vi "Create.vi"(5 "StringContains In":refnum<class "StringContains.lvclass">, 7 "Ignore Case (F)":bool, 8 "error in (no error)":errorcluster, 10 "Needle":string) -> (0 "error out":errorcluster, 3 "StringContains":refnum<class "StringContains.lvclass">)   [LabVIEW 2017, in "Transparent Assertions.lvlib" / "Constraints.lvlib" / "StringContains.lvclass"]
uses:
  StringContains.lvclass
  StringContains.lvclass/StringContains.ctl
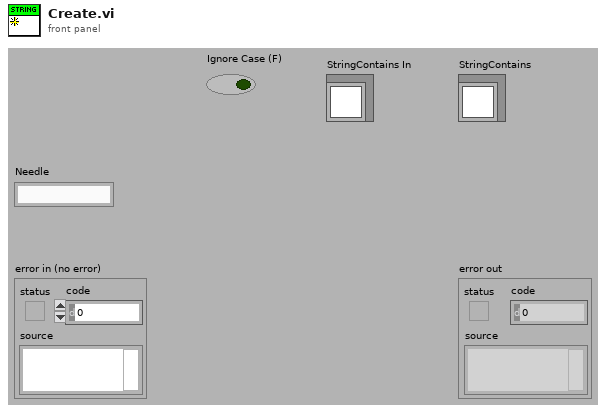
[diagram p1: front panel]
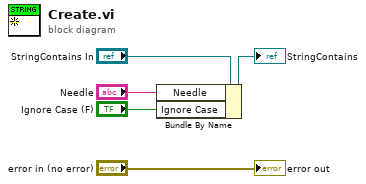
[diagram p0: block diagram]
diagram:
  n1 = Bundle By Name(cluster="StringContains In", "Needle"="Needle", "Ignore Case"="Ignore Case (F)") -> (→"StringContains":refnum<class "StringContains.lvclass">)
  "error out" <- "error in (no error)"
